vi "project.vi"() -> ()   [LabVIEW 2024]
uses:
  <vilib>/Analysis/4window.llb/windowTd.ctl
  <vilib>/numeric/Random Number (Range) DBL.vi
  <vilib>/measure/maspectr.llb/FFT Power Spectrum and PSD for 1 Chan.vi
  <vilib>/measure/NI_MAPro.lvlib
  <vilib>/Analysis/NI_AALPro.lvlib
  <vilib>/measure/NI_MABase.lvlib
panel:
  in  "stop":bool
  in  "Enum":enum16{"Sine", "Square", "Saw", "Noise"}(ring)=enum."Square"
  out "Waveform Graph 3":waveform(dbl)(graph)
  out "Waveform Graph 2":cluster{"f0":dbl, "df":dbl, "real part":dbl[]}(graph)
  in  "Slide":dbl(slide) scale=0.0..1000.0
  in  "choses x scale":i32(knob)=1 min=0 max=9 step=1 scale=0.0..6.0
  in  "frequency sample":dbl
  in  "signal freq":dbl
  # "44100 or 48000"
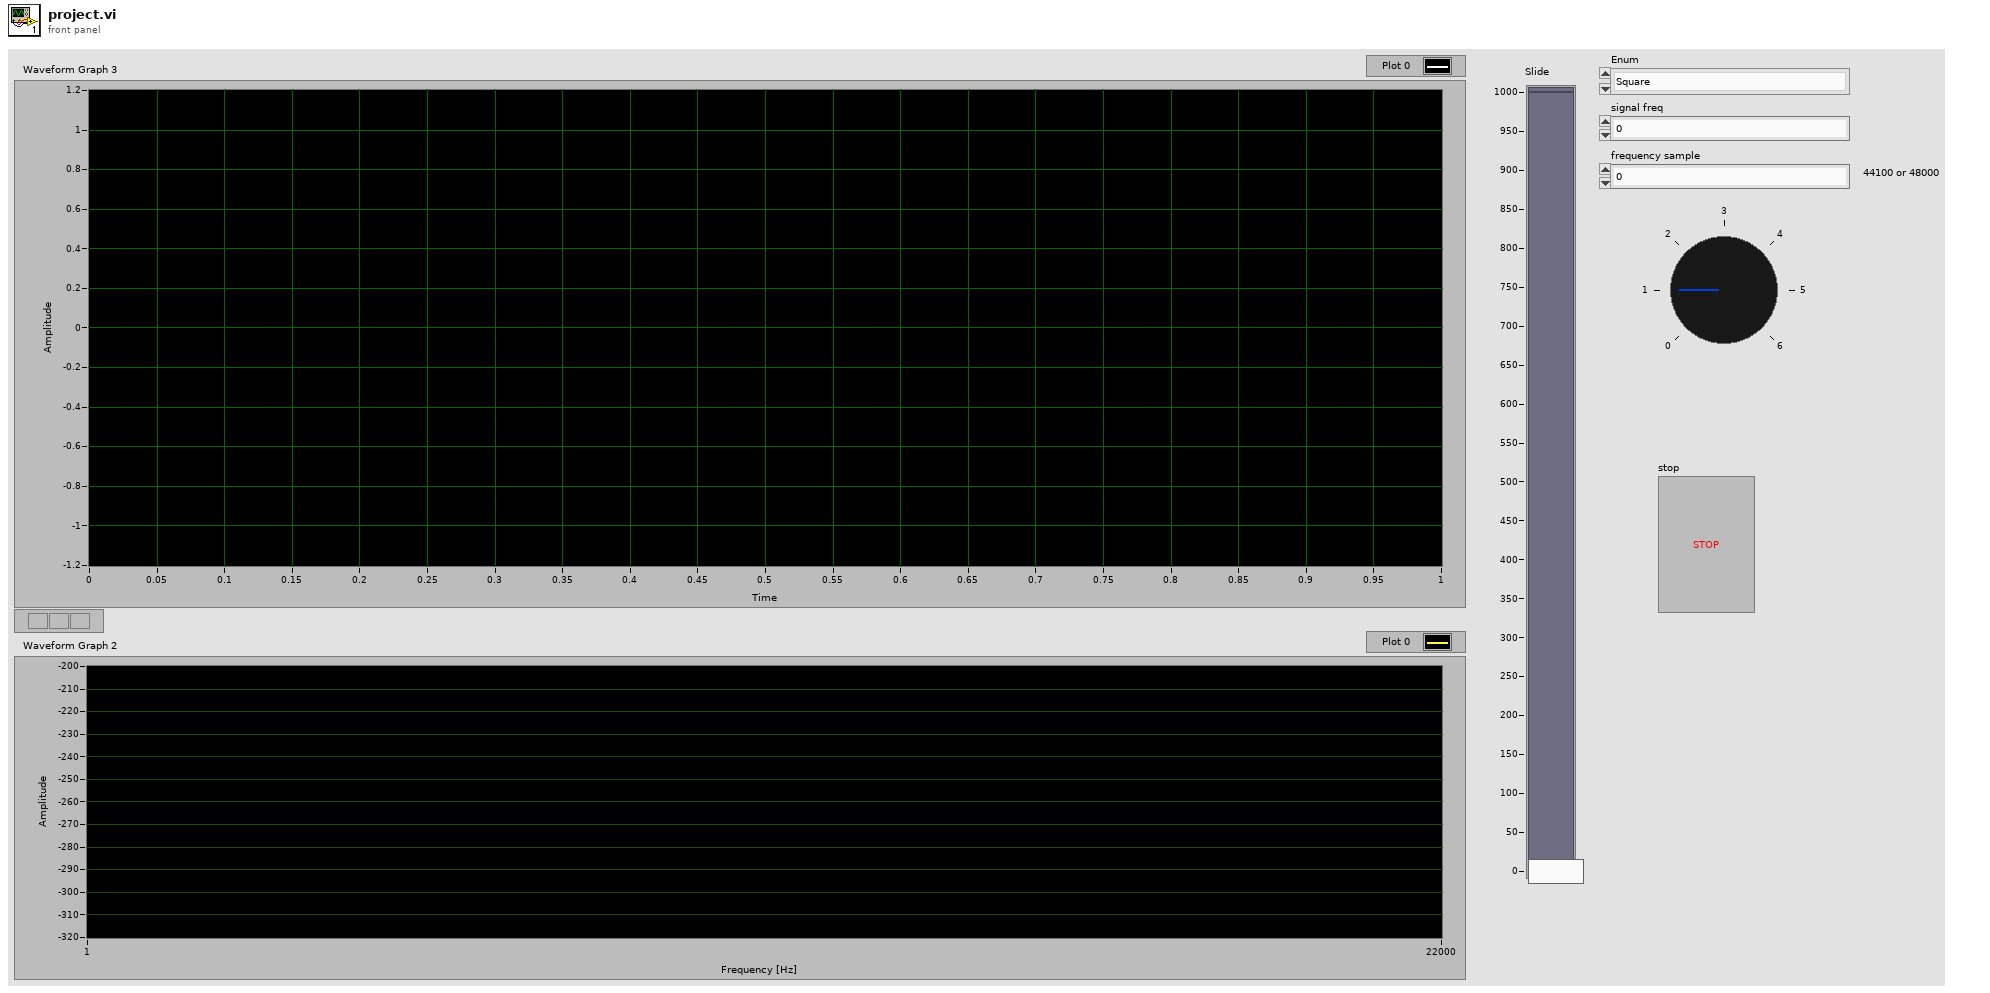
[diagram p1: front panel]
types:
  T1 = typedef "NI_AALPro.lvlib/windowTd.ctl" = u32
  T2 = cluster{"frequency sample":dbl, "frequency sample":dbl}
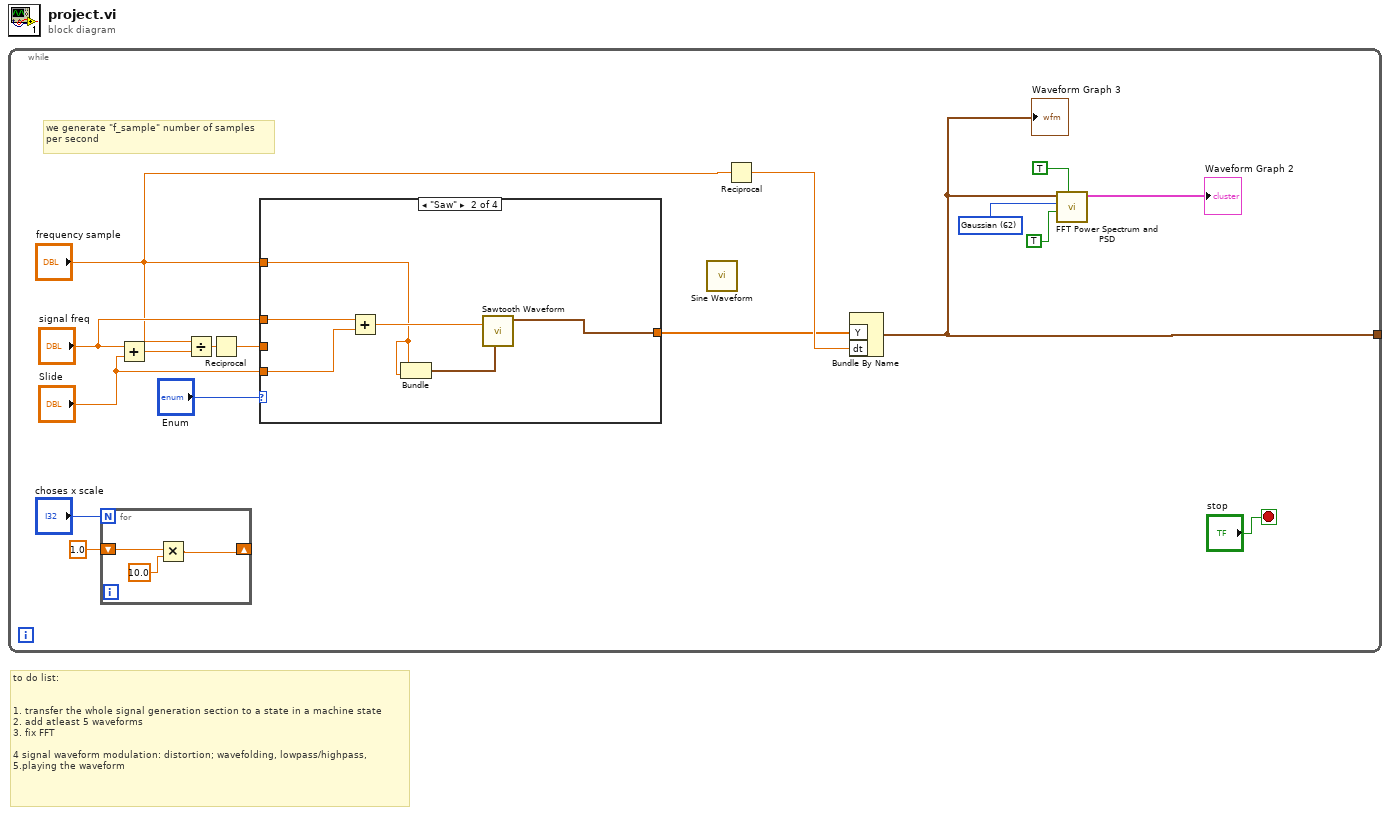
[diagram p0: block diagram]
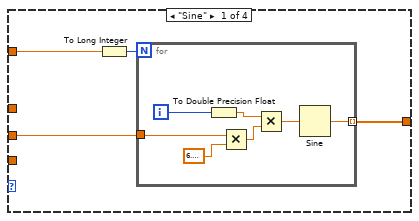
[diagram p2: hidden frame]
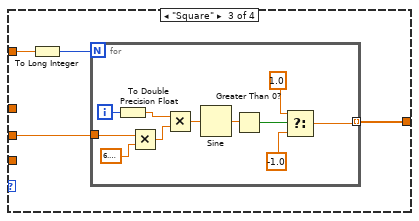
[diagram p3: hidden frame]
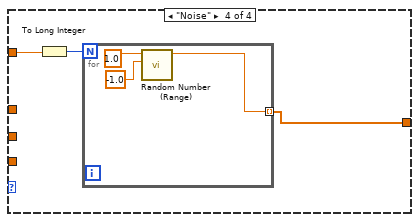
[diagram p4: hidden frame]
diagram:
  # "to do list:\n\n\n1. transfer the whole signal generation section to a state in a machine state\n2. add atleast 5 waveforms\n3. fix FFT\n\n4 signal waveform modulation: distortion; wavefolding, lowpass/highpass, \n5.playing the waveform"
  n1 = while {
    tunnel: [w1] -> _
    stop <- "stop" stop-if-true
    w10 = T1 62 items=["Rectangle"=0, "Hanning"=1, "Hamming"=2, "Blackman-Harris"=3, "Exact Blackman"=4, "Blackman"=5, "Flat Top"=6, "4 Term B-Harris "=7, "7 Term B-Harris"=8, "Low Sidelobe"=9, "Blackman Nuttall"=11, "Triangle"=30, "Bartlett-Hanning"=31, "Bohman"=32, "Parzen"=33, "Welch"=34, "Kaiser"=60, "Dolph-Chebyshev"=61, "Gaussian"=62] ("window")
    # "we generate \"f_sample\" number of samples per second"
    n2 = for {
      N: "choses x scale" -> [_]
      shift-right: [w56] -> _
      shift-left: 1.0 ("x") -> [w57]
      n3 = Multiply(x=w57, y=10.0) -> (x*y=w56:dbl)
    }
    n4 = Add(x="signal freq", y="Slide") -> (x+y=w15:dbl)
    n5 = Divide(x="frequency sample", y=w15) -> (x/y=w17:dbl)
    n6 = Reciprocal(x=w17) -> (1/x=w16:dbl)
    n7 = case shown="\"Saw\"" "Enum" {
      tunnel: [w21 w34 w38 w52] -> w2
      tunnel: w16 -> [w20 _ w37 _]
      tunnel: "signal freq" -> [_ w31 _ _]
      tunnel: "Slide" -> [_ w30 _ _]
      tunnel: "frequency sample" -> [w19 w29 w36 w51]
      frame "Sine" {
        n8 = To Long Integer(number=w19) -> (32bit integer=w18:i32)
        n9 = for {
          N: w18 -> [_]
          tunnel: [w22] -> w21 mode=indexing
          tunnel: w20 -> [w23]
          i -> [w26]
          n10 = To Double Precision Float(number=w26) -> (double precision float=w27:dbl)
          n11 = Multiply(x=w23, y=6.283185307179586) -> (x*y=w25:dbl)
          n12 = Multiply(x=w27, y=w25) -> (x*y=w28:dbl)
          n13 = Sine(x=w28) -> (sin(x)=w22:dbl)
        }
      }
      frame "Saw" {
        n14 = Add(x=w31, y=w30) -> (x+y=w32:dbl)
        n15 = Bundle("frequency sample"=w29, "frequency sample"=w29) -> (w33:T2)  [unwired: 1 in]
        n16 = call <vilib>:"Sawtooth Waveform.vi"("sampling info"=w33, "frequency"=w32) -> ("signal out"=w34:waveform(dbl))  [unwired: 8 in, 1 out]
      }
      frame "Square" {
        n17 = To Long Integer(number=w36) -> (32bit integer=w35:i32)
        n18 = for {
          N: w35 -> [_]
          tunnel: [w39] -> w38 mode=indexing
          tunnel: w37 -> [w44]
          i -> [w47]
          n19 = To Double Precision Float(number=w47) -> (double precision float=w48:dbl)
          n20 = Multiply(x=w44, y=6.283185307179586) -> (x*y=w46:dbl)
          n21 = Multiply(x=w48, y=w46) -> (x*y=w49:dbl)
          n22 = Sine(x=w49) -> (sin(x)=w43:dbl)
          n23 = Greater Than 0?(x=w43) -> (x > 0?=w42:bool)
          n24 = Select(t=1.0, s=w42, f=-1.0) -> (s? t:f=w39:dbl)
        }
      }
      frame "Noise" {
        n25 = To Long Integer(number=w51) -> (32bit integer=w50:i32)
        n26 = for {
          N: w50 -> [_]
          tunnel: [w53] -> w52 mode=indexing
          n27 = call-poly <vilib>:"Random Number (Range).vi"("lower bound (0)"=-1.0, "upper bound (100)"=1.0) -> ("number"=w53:dbl)  [unwired: 9 in]
        }
      }
    }
    n28 = call <vilib>:"Sine Waveform.vi"() -> ()  [unwired: 10 in, 2 out]
    n29 = Reciprocal(x="frequency sample") -> (1/x=w4:dbl)
    n30 = Bundle By Name("Y"=w2, "dt"=w4) -> (w1:waveform(dbl))  [unwired: 1 in]
    "Waveform Graph 3" <- w1
    n31 = call-poly <vilib>:"FFT Power Spectrum and PSD.vi"("restart averaging (F)"=TRUE, "dB On (F)"=TRUE, "window"=w10, "time signal"=w1) -> ("Power Spectrum / PSD"=→"Waveform Graph 2":cluster{"f0":dbl, "df":dbl, "magnitude":dbl[]})  [unwired: 4 in, 3 out]
  }
